vi "Odour_valve_pattern.vi"(4 "Pulse parameters":T1={"Conc. (ppm)"=10.0, "Pulse duration (ms)"=250.0, "Step duration (ms)"=2.0, "Sampling rate (Hz)"=20000.0, "Back valve ON delay (ms)"=-50.0, "Back valve OFF delay (ms)"=50.0, "VP (Hgmm)"=1.0} {"VP (Hgmm)" format="%#_13g"}) -> (0 "back valve pattern":bool[](array[boolean]), 1 "counter valve pattern":bool[](array[boolean]), 2 "odour valve pattern":bool[](array[boolean]))   [LabVIEW 2016]
uses:
  <vilib>/Waveform/DWDTOps.llb/DWDT Boolean Array to Digital.vi
panel:
  out "digital waveform":digitalwaveform(graph)
  out "Step delay duration (ms)":dbl=250.0 format="%#_13g"
  out "saturated VP (ppm)":dbl
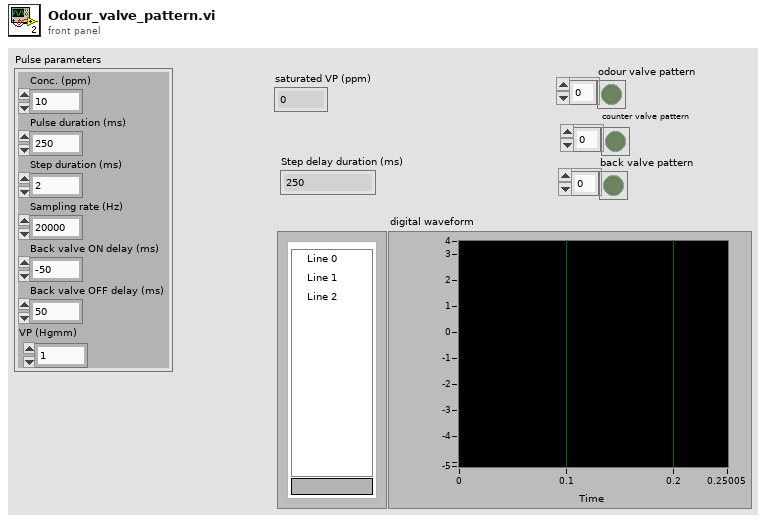
[diagram p1: front panel]
types:
  T1 = cluster{"Conc. (ppm)":dbl, "Pulse duration (ms)":dbl, "Step duration (ms)":dbl, "Sampling rate (Hz)":dbl, "Back valve ON delay (ms)":dbl, "Back valve OFF delay (ms)":dbl, "VP (Hgmm)":dbl}
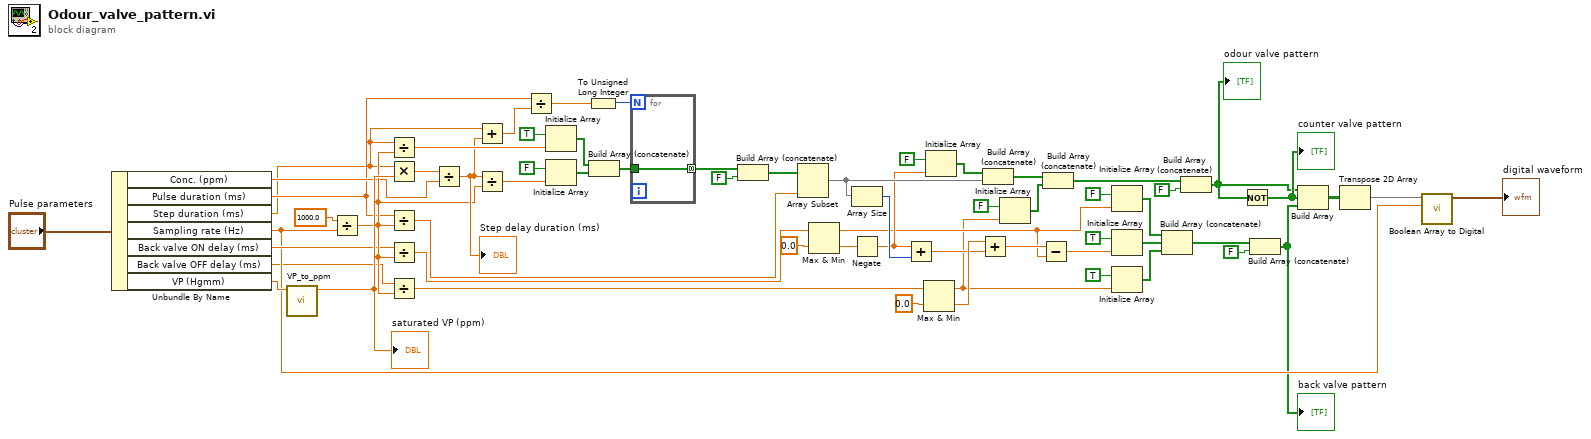
[diagram p0: block diagram]
diagram:
  n1 = Unbundle By Name("Pulse parameters") -> ("Conc. (ppm)"=w14:dbl, "Pulse duration (ms)"=w13:dbl, "Step duration (ms)"=w11:dbl, "Sampling rate (Hz)"=w9:dbl, "Back valve ON delay (ms)"=w10:dbl, "Back valve OFF delay (ms)"=w8:dbl, "VP (Hgmm)"=w12:dbl)
  n2 = call "VP_to_ppm.vi"("VP (Hgmm)"=w12) -> ("Saturated concentration (ppm)"=w62:dbl)  [unwired: 10 in]
  "saturated VP (ppm)" <- w62
  n3 = Divide(x=1000.0, y=w9) -> (x/y=w27:dbl)
  n4 = Divide(x=w11, y=w27) -> (x/y=w58:dbl)
  n5 = Multiply(x=w11, y=w62) -> (x*y=w61:dbl)
  n6 = Divide(x=w13, y=w27) -> (x/y=w48:dbl)
  n7 = Divide(x=w10, y=w27) -> (x/y=w34:dbl)
  n8 = Divide(x=w8, y=w27) -> (x/y=w29:dbl)
  n9 = Divide(x=w61, y=w14) -> (x/y=w53:dbl)
  "Step delay duration (ms)" <- w53
  n10 = Add(x=w11, y=w53) -> (x+y=w52:dbl)
  n11 = Divide(x=w53, y=w27) -> (x/y=w54:dbl)
  n12 = Divide(x=w13, y=w52) -> (x/y=w51:dbl)
  n13 = Initialize Array(TRUE, w58) -> (w57:bool[])
  n14 = Initialize Array(FALSE ("element"), w54) -> (w56:bool[])
  n15 = To Unsigned Long Integer(number=w51) -> (unsigned 32bit integer=w49:u32)
  n16 = Build Array (concatenate)(w57, w56) -> (w50:bool[])
  n17 = for {
    N: w49 -> [_]
    tunnel: w50 -> [w63]
    tunnel: [w63] -> w42 mode=concatenating
  }
  n18 = Build Array (concatenate)(w42, FALSE) -> (w37:bool[])
  n19 = Array Subset(array=w37, length=w48) -> (w33:bool[])  [unwired: 1 in]
  n20 = Max & Min(x=w34, y=0.0) -> (max(x,y)=w22:dbl, min(x,y)=w45:dbl)
  n21 = Array Size(array=w33) -> (size(s)=w36:i32)
  n22 = Negate(x=w45) -> (-x=w30:dbl)
  n23 = Add(x=w30, y=w36) -> (x+y=w25:dbl)
  n24 = Max & Min(x=w29, y=0.0) -> (max(x,y)=w17:dbl, min(x,y)=w26:dbl)
  n25 = Initialize Array(FALSE ("element"), w30) -> (w43:bool[])
  n26 = Add(x=w26, y=w25) -> (x+y=w23:dbl)
  n27 = Build Array (concatenate)(w43, w33) -> (w21:bool[])
  n28 = Initialize Array(FALSE ("element"), w17) -> (w19:bool[])
  n29 = Subtract(x=w23, y=w22) -> (x-y=w24:dbl)
  n30 = Build Array (concatenate)(w21, w19) -> (w6:bool[])
  n31 = Initialize Array(FALSE ("element"), w22) -> (w38:bool[])
  n32 = Initialize Array(TRUE ("element"), w24) -> (w35:bool[])
  n33 = Initialize Array(TRUE ("element"), w17) -> (w16:bool[])
  n34 = Build Array (concatenate)(w38, w35, w16) -> (w4:bool[])
  n35 = Build Array (concatenate)(w6, FALSE ("element")) -> (w1:bool[])
  "odour valve pattern" <- w1
  n36 = Not(x=w1) -> (.not. x?=w7:bool[])
  "counter valve pattern" <- w7
  n37 = Build Array (concatenate)(w4, FALSE ("element")) -> (w2:bool[])
  "back valve pattern" <- w2
  n38 = Build Array(w1, w7, w2) -> (w47:bool[][])
  n39 = Transpose 2D Array(2D array=w47) -> (transposed array=w32:bool[][])
  n40 = call-poly <vilib>:"Boolean Array to Digital.vi"("sample rate"=w9, "boolean array"=w32) -> ("digital waveform"=→"digital waveform":digitalwaveform)  [unwired: 8 in, 1 out]
